vi "Post-Build Action.vi"(5 "Files Generated by Build":path[](array[path]), 6 "Top Level/Always Included VIs":path[](array[path]), 7 "Destination Path":path, 8 "error in (no error)":errorcluster, 9 "Target Name":string, 10 "Build Specification Name":string, 11 "Project Path":path) -> (0 "error out":errorcluster)   [LabVIEW 2026]
uses:
  NationalInstruments.VeriStand
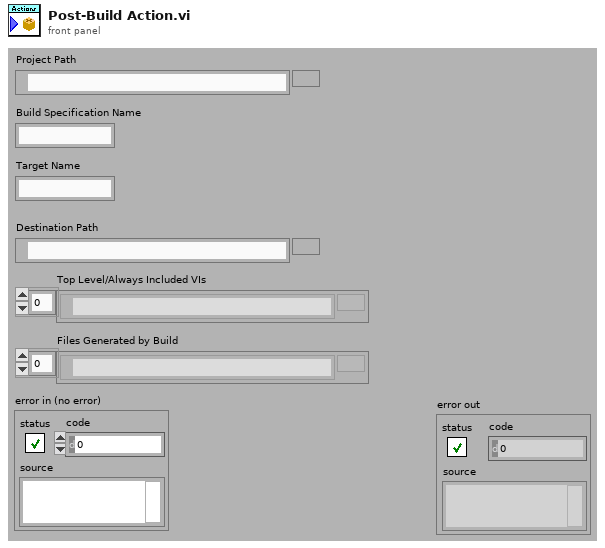
[diagram p1: front panel]
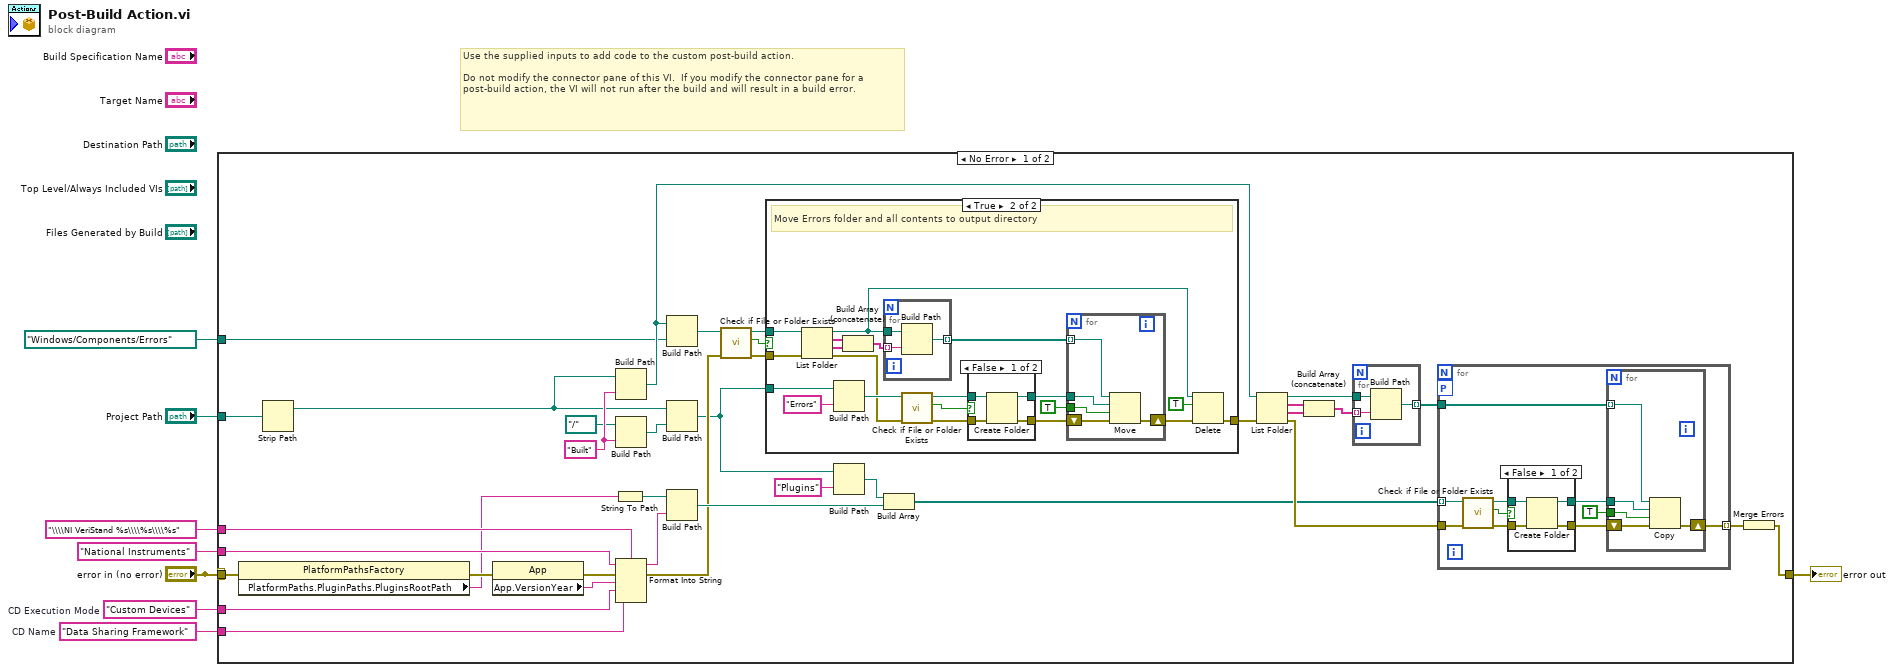
[diagram p0: block diagram]
diagram:
  w3 = "Data Sharing Framework"  # CD Name
  w4 = "Custom Devices"  # CD Execution Mode
  # "Use the supplied inputs to add code to the custom post-build action.\n\nDo not modify the connector pane of this VI.  If you modify the connector pane for a post-build action, the VI will not run after the build and will result in a build error."
  n1 = case shown="No Error" "error in (no error)" {
    selector: "error in (no error)" -> [_ w105]
    tunnel: [w24 w105] -> w8
    tunnel: "Project Path" -> [w38 _]
    tunnel: "\\\\NI VeriStand %s\\\\%s\\\\%s" ("name or relative path") -> [w30 _]
    tunnel: "National Instruments" ("name or relative path") -> [w29 _]
    tunnel: w4 -> [w28 _]
    tunnel: w3 -> [w27 _]
    tunnel: path "Windows/Components/Errors" ("base path") -> [w17 _]
    tunnel: "error in (no error)" -> [w11 _]
    frame No Error {
      w37 = "Built"
      n2 = property class="PlatformPathsFactory"(error in=w11) -> (error out=w12:errorcluster, "PlatformPaths.PluginPaths.PluginsRootPath"=w10:string)  [unwired: 1 in, 1 out]
      n3 = Strip Path(path=w38) -> (stripped path=w34:path)  [unwired: 1 out]
      n4 = property class="App"(error in=w12) -> (error out=w32:errorcluster, "App.VersionYear"=w33:string)  [unwired: 1 in, 1 out]
      n5 = String To Path(string=w10) -> (path=w9:path)
      n6 = Build Path(base path=w34, name or relative path=w37) -> (appended path=w18:path)
      n7 = Build Path(base path=path "../..", name or relative path=w37) -> (appended path=w36:path)
      n8 = Format Into String(format string=w30, initial string=w29, error in=w32, w33, w28, w27) -> (resulting string=w31:string, error out=w20:errorcluster)
      n9 = Build Path(base path=w18, name or relative path=w17) -> (appended path=w23:path)
      n10 = Build Path(base path=w34, name or relative path=w36) -> (appended path=w15:path)
      n11 = Build Path(base path=w9, name or relative path=w31) -> (appended path=w26:path)
      n12 = call <vilib>:"Check if File or Folder Exists.vi"("error in (no error)"=w20, "path"=w23) -> ("error out"=w21:errorcluster, "file or folder exists?"=w16:bool, "dup path"=w22:path)  [unwired: 7 in]
      n13 = case shown="True" w16 {
        tunnel: w22 -> [_ w66]
        tunnel: w15 -> [_ w55]
        tunnel: w21 -> [w46 w52]
        tunnel: [w46 w49] -> w19
        frame False {
          # "NO Errors folder, nothing to move"
        }
        frame True {
          # "Move Errors folder and all contents to output directory"
          n14 = List Folder(path=w66, error in=w52) -> (path out=w48:path, filenames=w63:string[], folder names=w62:string[], error out=w51:errorcluster)  [unwired: 2 in]
          n15 = Build Path(base path=w55, name or relative path="Errors") -> (appended path=w53:path)
          n16 = Build Array (concatenate)(w63, w62) -> (w64:string[])
          n17 = for {
            tunnel: w64 -> [w79] mode=indexing
            tunnel: w48 -> [w80]
            tunnel: [w78] -> w65 mode=indexing
            n18 = Build Path(base path=w80, name or relative path=w79) -> (appended path=w78:path)
          }
          n19 = call <vilib>:"Check if File or Folder Exists.vi"("error in (no error)"=w51, "path"=w53) -> ("error out"=w59:errorcluster, "file or folder exists?"=w61:bool, "dup path"=w60:path)  [unwired: 7 in]
          n20 = case shown="False" w61 {
            tunnel: w60 -> [w70 w72]
            tunnel: w59 -> [w69 w71]
            tunnel: [w68 w72] -> w58
            tunnel: [w67 w71] -> w57
            frame False {
              n21 = Create Folder(path (use dialog)=w70, error in=w69) -> (created path=w68:path, error out=w67:errorcluster)  [unwired: 1 in, 1 out]
            }
            frame True {
            }
          }
          n22 = for {
            tunnel: w65 -> [w75] mode=indexing
            shift-right: [w76] -> w50
            shift-left: w57 -> [w77]
            tunnel: w58 -> [w74]
            tunnel: TRUE ("overwrite (F)") -> [w73]
            n23 = Move(source path=w75, error in=w77, 9:w73, 10:w74) -> (error out=w76:errorcluster)  [unwired: 1 in, 2 out]
          }
          n24 = Delete(path (use dialog)=w48, entire hierarchy (F)=TRUE, error in=w50) -> (error out=w49:errorcluster)  [unwired: 2 in, 2 out]
        }
      }
      n25 = Build Path(base path=w15, name or relative path="Plugins") -> (appended path=w13:path)
      n26 = Build Array(w13, w26) -> (w25:path[])
      n27 = List Folder(path=w18, error in=w19) -> (path out=w45:path, filenames=w41:string[], folder names=w40:string[], error out=w43:errorcluster)  [unwired: 2 in]
      n28 = Build Array (concatenate)(w41, w40) -> (w39:string[])
      n29 = for {
        tunnel: w39 -> [w103] mode=indexing
        tunnel: w45 -> [w104]
        tunnel: [w102] -> w44 mode=indexing
        n30 = Build Path(base path=w104, name or relative path=w103) -> (appended path=w102:path)
      }
      n31 = for {
        tunnel: w44 -> [w87]
        workers-P: _ -> [_]
        tunnel: w25 -> [w81] mode=indexing
        tunnel: w43 -> [w86]
        tunnel: [w85] -> w42 mode=indexing
        n32 = call <vilib>:"Check if File or Folder Exists.vi"("error in (no error)"=w86, "path"=w81) -> ("error out"=w88:errorcluster, "file or folder exists?"=w90:bool, "dup path"=w89:path)  [unwired: 7 in]
        n33 = case shown="False" w90 {
          tunnel: w89 -> [w94 w96]
          tunnel: w88 -> [w93 w95]
          tunnel: [w92 w96] -> w84
          tunnel: [w91 w95] -> w83
          frame False {
            n34 = Create Folder(path (use dialog)=w94, error in=w93) -> (created path=w92:path, error out=w91:errorcluster)  [unwired: 1 in, 1 out]
          }
          frame True {
          }
        }
        n35 = for {
          tunnel: w87 -> [w99] mode=indexing
          shift-right: [w100] -> w85
          shift-left: w83 -> [w101]
          tunnel: w84 -> [w98]
          tunnel: TRUE ("overwrite (F)") -> [w97]
          n36 = Copy(8:w101, 9:w97, 10:w98, 11:w99) -> (0:w100:errorcluster)  [unwired: 1 in, 2 out]
        }
      }
      n37 = Merge Errors(w42) -> (w24:errorcluster)
    }
    frame Error {
    }
  }
  "error out" <- w8
